vi "ImgProc.vi"(5 "Optional Rectangle":i32[](array[numeric]), 7 "BCGTD":T2={"Brightness"=171.0, "Contrast"=55.999992, "Gamma"=2.0, "Threshold"=171.0, "Detection Sensitivity"=302.0, "Analyzing Speed"=10.0} {"Analyzing Speed" min=0.0 max=255.0 step=1.0 scale=0.0..255.0; "Detection Sensitivity" min=0 max=500 step=1 scale=0.0..500.0 scale format="%.2f"; "Threshold" min=0 max=255 step=1 scale=0.0..255.0 scale format="%.2f"; "Gamma" min=0.1 max=10 step=0.01 scale=0.1..10.0 scale format="%.1f"; "Contrast" min=1 max=89 step=0.1 scale=30.0..60.0 scale format="%.2f"; "Brightness" min=0 max=255 step=1 scale=0.0..255.0 scale format="%.2f"}, 10 "Image Dst":T1, 11 "Image Src":T1) -> (2 "Particle Measurements (Pixels)":dbl[][](array[numeric]) format="%.2f", 3 "Image Out (duplicate)":T1)   [LabVIEW 2012]
uses:
  <vilib>/vision/Image Controls.llb/IMAQ Image.ctl
  <vilib>/Utility/error.llb/DialogType.ctl
  <vilib>/vision/NI_Vision_Development_Module.lvlib
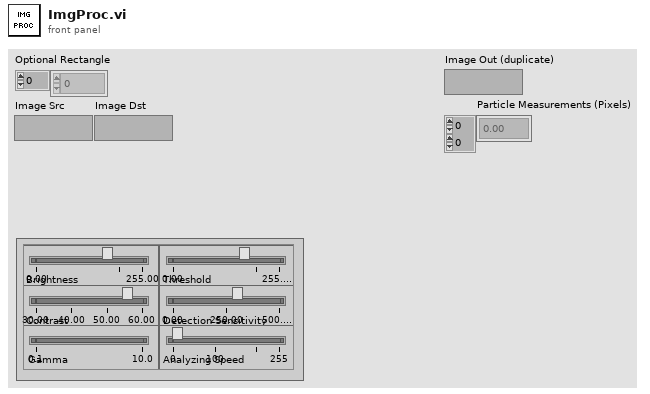
[diagram p1: front panel]
types:
  T1 = typedef "IMAQ Image.ctl" = refnum<image>
  T2 = cluster{"Brightness":sgl, "Contrast":sgl, "Gamma":sgl, "Threshold":sgl, "Detection Sensitivity":sgl, "Analyzing Speed":dbl}
  T3 = typedef "DialogType.ctl" = u16
  T4 = typedef "Particle Parameters" = i32
  T5 = cluster{"Measurement Parameter":T4, "Range Lower Value":dbl, "Range Upper Value":dbl, "Range":bool, "Measurement Type":bool}[]
  T6 = cluster{"Brightness":sgl, "Contrast":sgl, "Gamma":sgl}
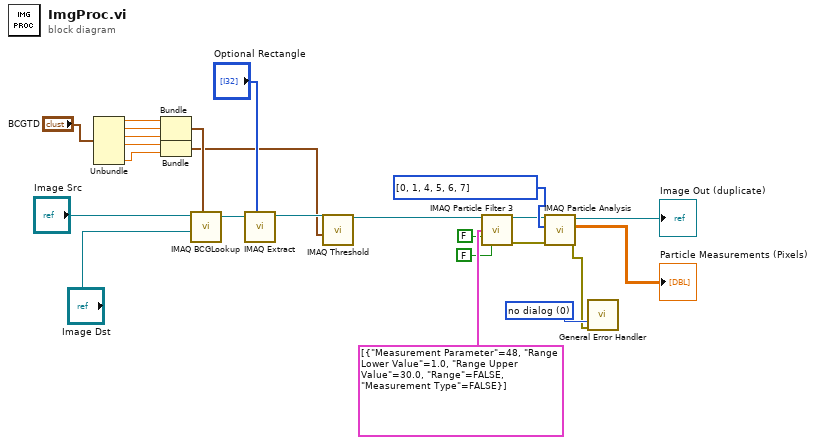
[diagram p0: block diagram]
diagram:
  w23 = T3 0 items=["no dialog", "OK message", "continue or stop message", "OK message + warnings", "continue/stop + warnings"] ("type of dialog (OK msg:1)")
  w20 = T4[] [0, 1, 4, 5, 6, 7] items=["Center of Mass X", "Center of Mass Y", "First Pixel X", "First Pixel Y", "Bounding Rect Left", "Bounding Rect Top", "Bounding Rect Right", "Bounding Rect Bottom", "Max Feret Diameter Start X", "Max Feret Diameter Start Y", "Max Feret Diameter End X", "Max Feret Diameter End Y", "Max Horiz. Segment Length Left", "Max Horiz. Segment Length Right", "Max Horiz. Segment Length Row", "-", "Bounding Rect Width", "Bounding Rect Height", "Bounding Rect Diagonal", "Perimeter", "Convex Hull Perimeter", "Holes' Perimeter", "Max Feret Diameter", "Equivalent Ellipse Major Axis", "Equivalent Ellipse Minor Axis", "Equivalent Ellipse Minor Axis (Feret)", "Equivalent Rect Long Side", "Equivalent Rect Short Side", "Equivalent Rect Diagonal", "Equivalent Rect Short Side (Feret)", "Average Horiz. Segment Length", "Average Vert. Segment Length", "Hydraulic Radius", "Waddel Disk Diameter", "-", "Area", "Holes' Area", "Particle & Holes' Area", "Convex Hull Area", "Image Area", "-", "Number of Holes", "Number of Horiz. Segments", "Number of Vert. Segments", "-", "Orientation", "Max Feret Diameter Orientation", "-", "% Area/Image Area", "% Area/(Particle & Holes' Area)", "Ratio of Equivalent Ellipse Axes", "Ratio of Equivalent Rect Sides", "-", "Elongation Factor", "Compactness Factor", "Heywood Circularity Factor", "Type Factor", "-", "Sum X", "Sum Y", "Sum XX", "Sum XY", "Sum YY", "Sum XXX", "Sum XXY", "Sum XYY", "Sum YYY", "-", "Moment of Inertia XX", "Moment of Inertia XY", "Moment of Inertia YY", "Moment of Inertia XXX", "Moment of Inertia XXY", "Moment of Inertia XYY", "Moment of Inertia YYY", "Norm. Moment of Inertia XX", "Norm. Moment of Inertia XY", "Norm. Moment of Inertia YY", "Norm. Moment of Inertia XXX", "Norm. Moment of Inertia XXY", "Norm. Moment of Inertia XYY", "Norm. Moment of Inertia YYY", "Hu Moment 1", "Hu Moment 2", "Hu Moment 3", "Hu Moment 4", "Hu Moment 5", "Hu Moment 6", "Hu Moment 7"] ("Pixel Measurements")
  n1 = Unbundle("BCGTD") -> ("Brightness"=w11:sgl, "Contrast"=w10:sgl, "Gamma"=w9:sgl, "Threshold"=w7:sgl, "Analyzing Speed"=w5:dbl)  [unwired: 1 out]
  n2 = Bundle("Brightness"=w11, "Contrast"=w10, "Gamma"=w9) -> (w8:T6)  [unwired: 1 in]
  n3 = Bundle("Threshold"=w7, "Analyzing Speed"=w5) -> (w6:cluster{"Threshold":sgl, "Analyzing Speed":dbl})  [unwired: 1 in]
  n4 = call "IMAQ BCGLookup"("Image Src"="Image Src", "BCG Values"=w8, "Image Dst"="Image Dst") -> ("Image Dst Out"=w16:T1)  [unwired: 4 in, 1 out]
  n5 = call "IMAQ Extract"("Optional Rectangle"="Optional Rectangle", "Image Src"=w16) -> ("Image Dst Out"=w24:T1)  [unwired: 4 in, 5 out]
  n6 = call "IMAQ Threshold"("Range"=w6, "Image Src"=w24) -> ("Image Dst Out"=w1:T1)  [unwired: 8 in, 1 out]
  n7 = call "IMAQ Particle Filter 3"("Image Src"=w1, "Selection Values"=T5 [{"Measurement Parameter"=48, "Range Lower Value"=1.0, "Range Upper Value"=30.0, "Range"=FALSE, "Measurement Type"=FALSE}], "Keep/Remove Particles (F)"=FALSE, "Reject Border? (F)"=FALSE) -> ("Image Dst Out"=w19:T1, "error out"=w3:errorcluster)  [unwired: 5 in, 5 out]
  n8 = call "IMAQ Particle Analysis"("error in (no error)"=w3, "Pixel Measurements"=w20, "Image"=w19) -> ("error out"=w2:errorcluster, "Particle Measurements (Pixels)"=→"Particle Measurements (Pixels)":dbl[][], "Image Out (duplicate)"=→"Image Out (duplicate)":T1)  [unwired: 3 in, 3 out]
  n9 = call <vilib>:"General Error Handler.vi"("type of dialog (OK msg:1)"=w23, "error in (no error)"=w2) -> ()  [unwired: 9 in, 5 out]
